vi "resetStiffnessData.vi"(8 "error in (no error)":errorcluster, 11 "Model in":refnum<class "Model.lvclass">) -> (0 "error out":errorcluster, 3 "Model out":refnum<class "Model.lvclass">)   [LabVIEW 2015, in "Model.lvclass"]
uses:
  Model.lvclass
  Model.lvclass/Model.ctl
  ApplicationElements/StiffnessCalculator/StiffnessCalculator.lvclass
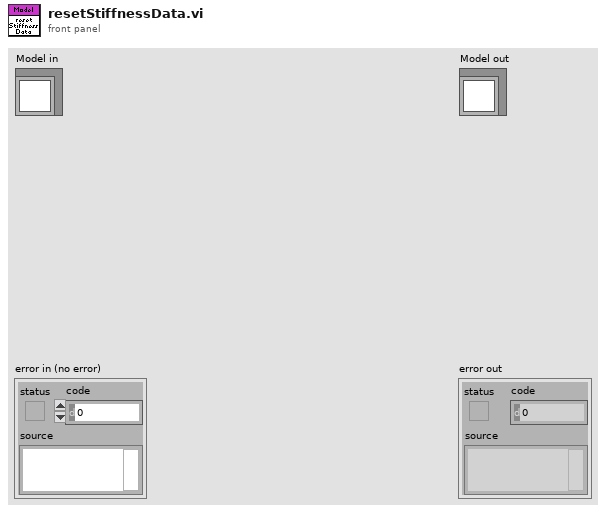
[diagram p1: front panel]
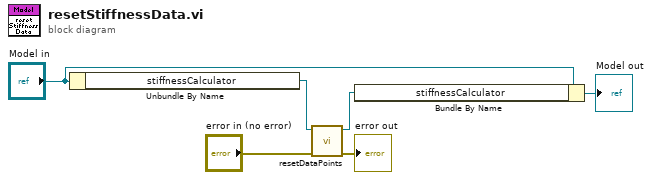
[diagram p0: block diagram]
diagram:
  n1 = Unbundle By Name("Model in") -> ("stiffnessCalculator"=w4:refnum<class "StiffnessCalculator.lvclass">)
  n2 = call "resetDataPoints.vi"("error in (no error)"="error in (no error)", "StiffnessCalculator in"=w4) -> ("error out"=→"error out":errorcluster, "StiffnessCalculator out"=w3:refnum<class "StiffnessCalculator.lvclass">)  [unwired: 8 in]
  n3 = Bundle By Name(cluster="Model in", "stiffnessCalculator"=w3) -> (→"Model out":refnum<class "Model.lvclass">)
